vi "Test_Copy_Raw_Memory_To_Image_ARGB.vi"(8 "error in (no error)":errorcluster, 11 "Test Case In":refnum<class "Image.lvclass">) -> (0 "error out":errorcluster, 3 "Test Case Out":refnum<class "Image.lvclass">)   [LabVIEW 2020, in "g_ar_toolkit.test.lvlib" / "Image.lvclass"]
uses:
  Image.lvclass
  Image.lvclass/Image.ctl
  g_ar_toolkit.image/Image Size (Fixed).ctl
  g_ar_toolkit.image/g_ar_toolkit.image.lvlib
  g_ar_toolkit.image/CreateEmptyImageARGB.vi
  g_ar_toolkit.image/Raw Memory Information Dimension.ctl
  g_ar_toolkit.image/Raw Memory Information.ctl
  4993e8ee-a06a-463a-9684-69129f64d5ce.vi
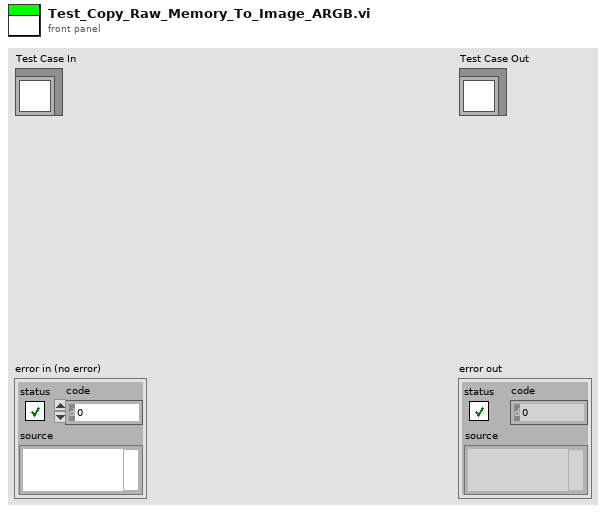
[diagram p1: front panel]
types:
  T1 = typedef "g_ar_toolkit.image.lvlib/Image Size (Fixed).ctl" = cluster{"Width":u16, "Height":u16}
  T2 = typedef "imagedata.ctl" = cluster{"image type":i32, "image depth":i32, "image":u8[], "mask":u8[], "colors":u32[], "Rectangle":cluster{"left":i16, "top":i16, "right":i16, "bottom":i16}}
  T3 = typedef "g_ar_toolkit.image.lvlib/Raw Memory Information.ctl" = cluster{"Memory Address":u64, "Dimension 0":T4, "Dimension 1":T4}
  T4 = typedef "g_ar_toolkit.image.lvlib/Raw Memory Information Dimension.ctl" = cluster{"Size":u16, "Stride":u32}
  T5 = cluster{"pointer":u64, "size_0":u32, "stride_0":i32, "size_1":u32, "stride_1":i32, "element size":u32, "subarray?":bool}
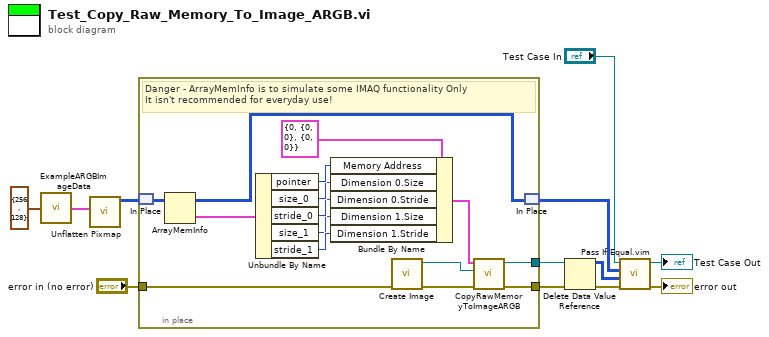
[diagram p0: block diagram]
diagram:
  n1 = call "ExampleARGBImageData.vi"("Image Size"=T1 {"Width"=256, "Height"=128}) -> ("RGB Image Data"=w4:T2)
  n2 = call <vilib>:"Unflatten Pixmap.vi"("image data"=w4) -> ("24-bit pixmap"=w2:u32[][])  [unwired: 4 in, 6 out]
  n3 = in-place {
    in-place-border: [w18] -> w9
    in-place-border: "error in (no error)" -> [w16]
    in-place-border: [w15] -> w6
    # "Danger - ArrayMemInfo is to simulate some IMAQ functionality Only\nIt isn't recommended for everyday use!"
    n4 = in-place-match #1(w2) -> (w14:u32[][])
    n5 = ArrayMemInfo(3:w14) -> (0:w27:T5, 1:w13:u32[][])
    n6 = Unbundle By Name(w27) -> ("pointer"=w26:u64, "size_0"=w24:u32, "stride_0"=w23:i32, "size_1"=w21:u32, "stride_1"=w22:i32)
    n7 = Bundle By Name(cluster=T3 {"Memory Address"=0, "Dimension 0"={"Size"=0, "Stride"=0}, "Dimension 1"={"Size"=0, "Stride"=0}} ("Source"), "Memory Address"=w26, "Dimension 0.Size"=w24, "Dimension 0.Stride"=w23, "Dimension 1.Size"=w21, "Dimension 1.Stride"=w22) -> (w19:T3)
    n8 = call-poly "Create Image.vi"("error in (no error)"=w16) -> ("error out"=w17:errorcluster, "New ARGB Image"=w25:refnum<data-value>)  [unwired: 9 in]
    n9 = call "CopyRawMemoryToImageARGB.vi"("error in (no error)"=w17, "ARGB Image Destination"=w25, "Source"=w19) -> ("error out"=w15:errorcluster, "ARGB Image Destination (Duplicate)"=w18:refnum<data-value>)  [unwired: 7 in]
    n10 = in-place-match #1(w13) -> (w1:u32[][])
  }
  n11 = Delete Data Value Reference(data value reference=w9, error in=w6) -> (data value=w8:u32[][], error out=w5:errorcluster)
  n12 = call "Pass If Equal.vim"("error in (no error)"=w5, "Actual"=w8, "Expected"=w1, "LUnit Test Case In"="Test Case In") -> ("error out"=→"error out":errorcluster, "LUnit Test Case Out"=→"Test Case Out":refnum<class "Image.lvclass">)  [unwired: 6 in]
